vi "SetFont.vi"(8 "error in (no error)":errorcluster, 10 "font":cluster{"name":string, "size":i16, "color":u32}, 11 "menu in":refnum<class "menu.lvclass">) -> (0 "error out":errorcluster, 3 "menu out":refnum<class "menu.lvclass">)   [LabVIEW 2009, in "menu.lvclass"]
uses:
  menu.lvclass
  menu.lvclass/menu.ctl
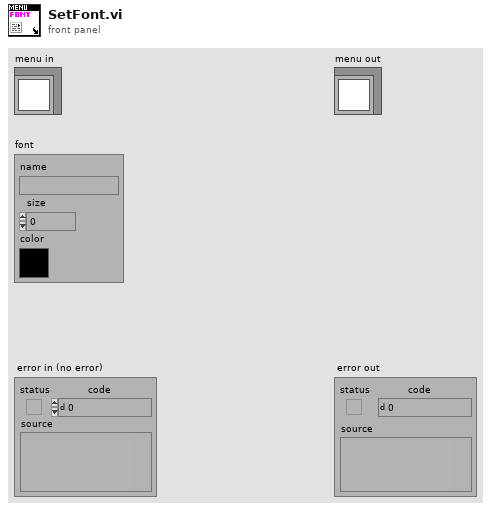
[diagram p1: front panel]
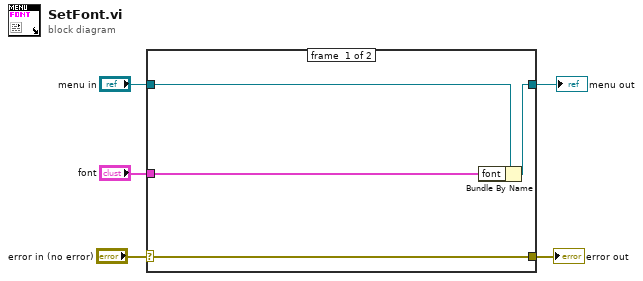
[diagram p0: block diagram]
diagram:
  n1 = case shown="No Error" "error in (no error)" {
    selector: "error in (no error)" -> [w9 w10]
    tunnel: [w9 w10] -> w2
    tunnel: [w7 w11] -> w4
    tunnel: "menu in" -> [w8 w11]
    tunnel: "font" -> [w6 _]
    frame #0 {
      n2 = Bundle By Name(cluster=w8, "font"=w6) -> (w7:refnum<class "menu.lvclass">)
    }
    frame #1 {
    }
  }
  "error out" <- w2
  "menu out" <- w4
